vi "Dequeue Message.vi"(8 "error in (no error)":T1 caption="Fehler (Eingang, kein Fehler)", 11 "Nachrichten-Queue":refnum<queue>) -> (0 "error out":T1 caption="Fehler (Ausgang)", 1 "Nachrichtendaten":variant, 2 "Nachricht":string, 3 "Nachrichten-Queue (Kopie)":refnum<queue>)   [LabVIEW 2014, in "MyQH Message Queue.lvlib"]
doc: "Dieses VI entfernt Nachrichten aus der Nachrichten-Queue."
uses:
  MyQH Message Queue.lvlib
  Message Cluster.ctl
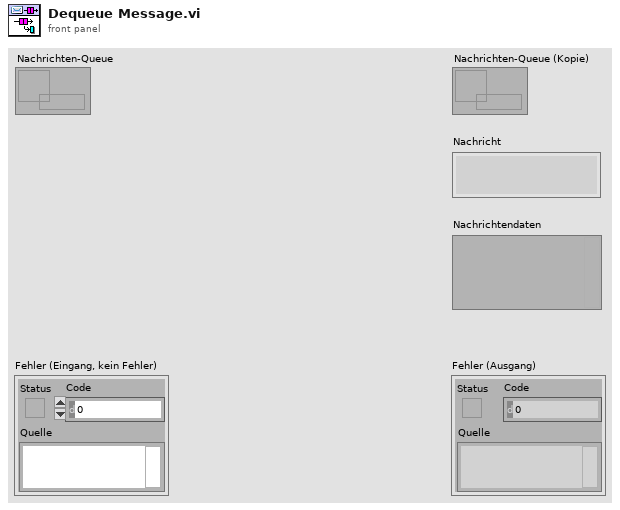
[diagram p1: front panel]
types:
  T1 = cluster{"Status":bool, "Code":i32, "Quelle":string}
  T2 = typedef "MyQH Message Queue.lvlib/Message Cluster.ctl" = cluster{"Nachricht":string, "Nachrichtendaten":variant}
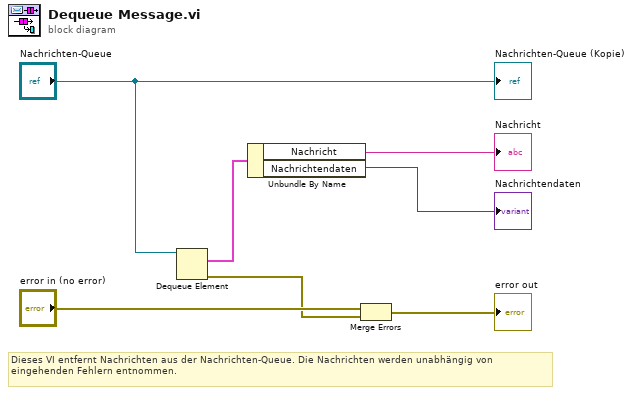
[diagram p0: block diagram]
diagram:
  # "Dieses VI entfernt Nachrichten aus der Nachrichten-Queue. Die Nachrichten werden unabhängig von eingehenden Fehlern entnommen."
  n1 = Dequeue Element(queue="Nachrichten-Queue") -> (element=w4:T2, error out=w1:errorcluster)  [unwired: 2 in, 2 out]
  n2 = Unbundle By Name(w4) -> ("Nachricht"=→"Nachricht":string, "Nachrichtendaten"=→"Nachrichtendaten":variant)
  n3 = Merge Errors("error in (no error)", w1) -> (→"error out":errorcluster)
  "Nachrichten-Queue (Kopie)" <- "Nachrichten-Queue"
